vi "变量.vi"(7 "write":cluster{"VISA":bool, "COM":bool}, 10 "COM":bool=TRUE, 11 "VISA resource in":refnum<visa-resource-name>) -> (2 "COM out":bool, 3 "VISA resource out":refnum<visa-resource-name>)   [LabVIEW 2016]
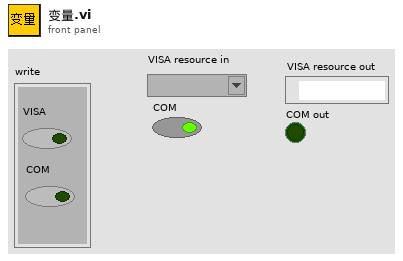
[diagram p1: front panel]
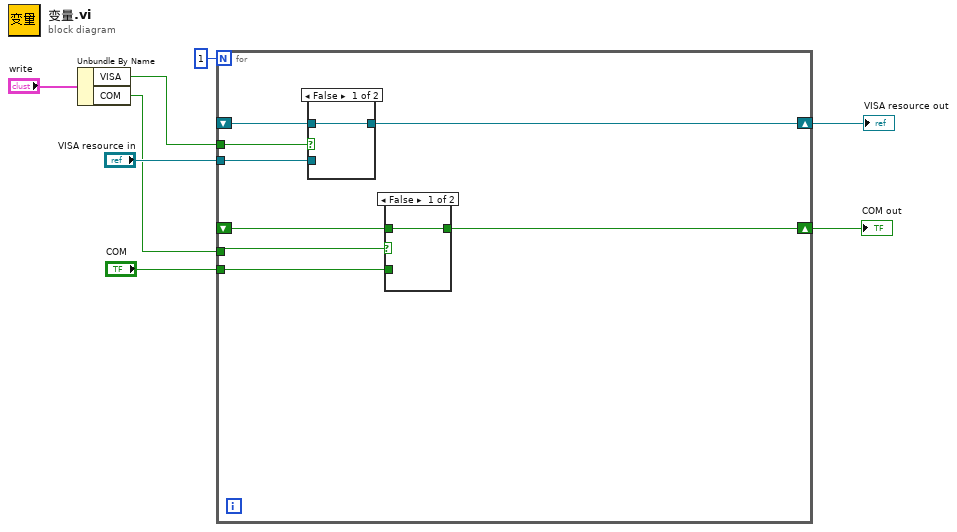
[diagram p0: block diagram]
diagram:
  n1 = Unbundle By Name("write") -> ("VISA"=w1:bool, "COM"=w2:bool)
  n2 = for {
    N: 1 -> [_]
    shift-right: [w15] -> w7
    shift-left: _ -> [w14]
    tunnel: "VISA resource in" -> [w16]
    shift-right: [w12] -> w4
    shift-left: _ -> [w11]
    tunnel: "COM" -> [w13]
    tunnel: w2 -> [w10]
    tunnel: w1 -> [w9]
    n3 = case shown="False" w9 {
      tunnel: w16 -> [_ w20]
      tunnel: [w19 w20] -> w15
      tunnel: w14 -> [w19 _]
      frame False {
      }
      frame True {
      }
    }
    n4 = case shown="False" w10 {
      tunnel: w13 -> [_ w18]
      tunnel: [w17 w18] -> w12
      tunnel: w11 -> [w17 _]
      frame False {
      }
      frame True {
      }
    }
  }
  "VISA resource out" <- w7
  "COM out" <- w4
